vi "CRYDB Connect Through UDL DSN.vi"(11 "DB Path":path) -> (0 "error out":errorcluster, 2 "bResult":bool, 3 "connection reference":T1)   [LabVIEW 2013]
uses:
  <vilib>/addons/database/Connection.llb/Conn ObjectReference.ctl
  <vilib>/addons/database/Connection.llb/DB Tools Open Connec (String).vi
  <vilib>/addons/database/Connection.llb/DB Tools Open Connec (Path).vi
  <vilib>/addons/database/NI_Database_API.lvlib
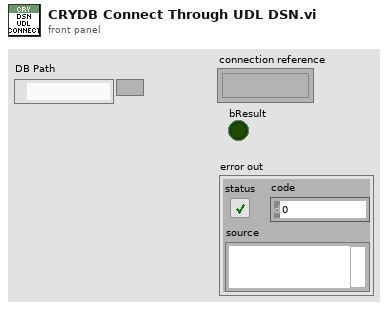
[diagram p1: front panel]
types:
  T1 = typedef "NI_Database_API.lvlib/Conn ObjectReference.ctl" = refnum<k1>
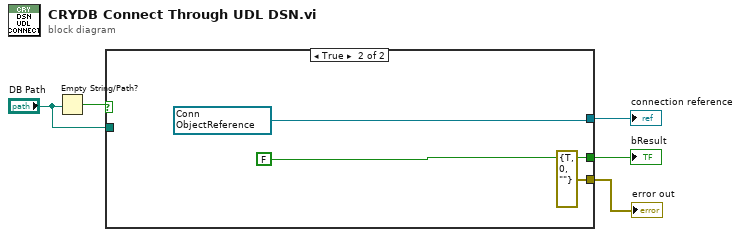
[diagram p0: block diagram]
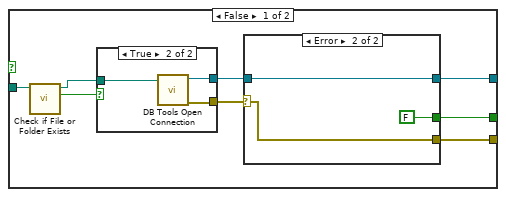
[diagram p2: hidden frame]
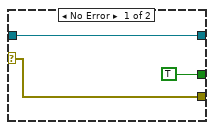
[diagram p3: hidden frame]
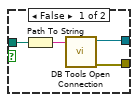
[diagram p4: hidden frame]
diagram:
  n1 = Empty String/Path?(string/path="DB Path") -> (empty?=w5:bool)
  n2 = case shown="True" w5 {
    tunnel: "DB Path" -> [w13 _]
    tunnel: [w8 w29] -> w2
    tunnel: [w7 FALSE] -> w3
    tunnel: [w6 errorcluster {"status"=TRUE, "code"=0, "source"=""} ("error IO")] -> w1
    frame False {
      n3 = call <vilib>:"Check if File or Folder Exists.vi"("path"=w13) -> ("file or folder exists?"=w12:bool, "dup path"=w11:path)  [unwired: 8 in, 1 out]
      n4 = case shown="True" w12 {
        tunnel: w11 -> [w23 w26]
        tunnel: [w21 w25] -> w9
        tunnel: [w20 w24] -> w10
        frame False {
          n5 = Path To String(path=w23) -> (string=w22:string)
          n6 = call-poly <vilib>:"DB Tools Open Connection.vi"("connection information"=w22) -> ("error out"=w20:errorcluster, "connection reference"=w21:T1)  [unwired: 7 in]
        }
        frame True {
          n7 = call-poly <vilib>:"DB Tools Open Connection.vi"("connection information"=w26) -> ("error out"=w24:errorcluster, "connection reference"=w25:T1)  [unwired: 7 in]
        }
      }
      n8 = case shown="Error" w10 {
        selector: w10 -> [w14 w17]
        tunnel: w9 -> [w16 w18]
        tunnel: [w16 w18] -> w8
        tunnel: [TRUE FALSE] -> w7
        tunnel: [w14 w17] -> w6
        frame No Error {
        }
        frame Error {
        }
      }
    }
    frame True {
      w29 = T1 refnum items=["Connection"] ("connection reference")
    }
  }
  "bResult" <- w3
  "connection reference" <- w2
  "error out" <- w1
